vi "TCPIP RED WRITE.vi"() -> ()   [LabVIEW 2015]
uses:
  Galobal variable_TI.vi
panel:
  out "NG":bool
  out "Ok":bool
  out "loop Itration":i32
  out "Coordinate":string
  out "Data Read":string
  out "substring":string
  in  "Data Write":string
  out "data out 2":string
  out "error out 3":errorcluster
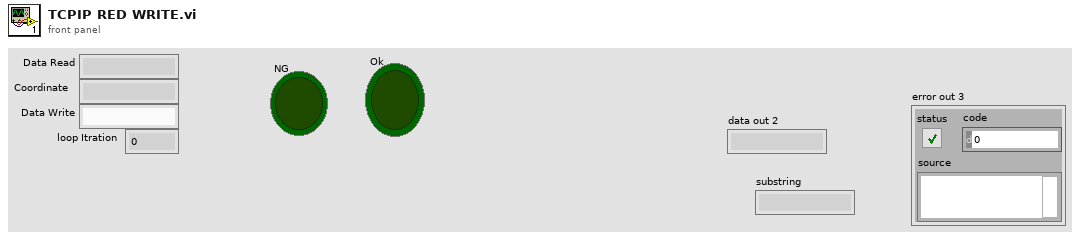
[diagram p1: front panel]
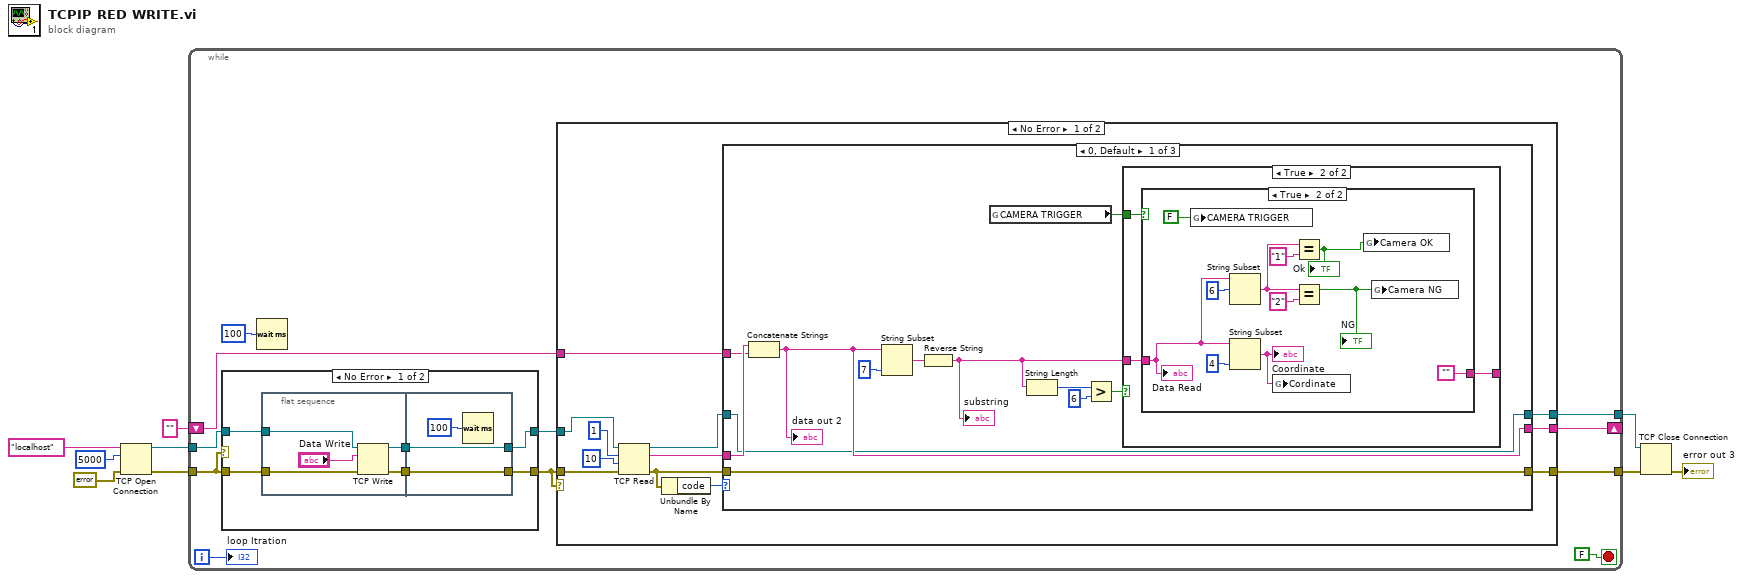
[diagram p0: block diagram]
diagram:
  n1 = TCP Open Connection(address="localhost", remote port or service name=u16 5000, error in (no error)=errorcluster {"status"=FALSE, "code"=0, "source"=""}) -> (connection ID=w3:refnum<k5>, error out=w2:errorcluster)  [unwired: 2 in]
  n2 = while {
    tunnel: [w18] -> w8
    tunnel: [w17] -> w7
    tunnel: w3 -> [w14]
    tunnel: w2 -> [w11]
    shift-right: [w15] -> _
    shift-left: "" -> [w16]
    i -> [w10]
    stop <- FALSE stop-if-true
    n3 = case shown="No Error" w11 {
      tunnel: w14 -> [w26 w36]
      tunnel: w11 -> [w25 w35]
      tunnel: [w24 w36] -> w12
      tunnel: [w23 w35] -> w13
      frame No Error {
        n4 = flat-sequence {
          tunnel: w26 -> [w31]
          tunnel: w25 -> [w30]
          tunnel: [w29] -> w22
          tunnel: [w28] -> w21
          tunnel: [w33] -> w23
          tunnel: [w34] -> w24
          tunnel: w22 -> [w34]
          tunnel: w21 -> [w33]
          frame #0 {
            n5 = TCP Write(connection ID=w31, data in="Data Write", error in (no error)=w30) -> (connection ID out=w29:refnum<k5>, error out=w28:errorcluster)  [unwired: 1 in, 1 out]
          }
          frame #1 {
            n6 = Wait (ms)(milliseconds to wait=u32 100) -> ()  [unwired: 1 out]
          }
        }
      }
      frame Error {
      }
    }
    n7 = Wait (ms)(milliseconds to wait=u32 100) -> ()  [unwired: 1 out]
    n8 = case shown="No Error" w13 {
      tunnel: [w39 w83] -> w18
      tunnel: [w37 w82] -> w17
      tunnel: w12 -> [w46 w83]
      tunnel: w13 -> [w45 w82]
      tunnel: w16 -> [w43 w81]
      tunnel: [w42 w81] -> w15
      frame No Error {
        n9 = TCP Read(connection ID=w46, bytes to read=1, error in (no error)=w45, 9:10 ("timeout ms (25000)")) -> (connection ID out=w40:refnum<k5>, data out=w44:string, error out=w38:errorcluster)  [unwired: 1 in]
        n10 = Unbundle By Name(w38) -> ("code"=w41:i32)
        n11 = case shown="0, Default" w41 {
          tunnel: w44 -> [w60 _ w79]
          tunnel: w43 -> [w59 w78 _]
          tunnel: [w58 w78 w79] -> w42
          tunnel: [w50 w77 w80] -> w39
          tunnel: w40 -> [w50 w77 w80]
          tunnel: w38 -> [w49 _ _]
          tunnel: [w49 _ _] -> w37
          frame 0, Default {
            n12 = Concatenate Strings(w60, w59) -> (w58:string)
            "data out 2" <- w58
            n13 = String Subset(string=w58, length (rest)=7 ("length (rest)")) -> (substring=w56:string)  [unwired: 1 in]
            n14 = Reverse String(1:w56) -> (0:w51:string)
            "substring" <- w51
            n15 = global read "Galobal variable_TI.vi" "CAMERA TRIGGER"() -> (w53:bool)
            n16 = String Length(string=w51) -> (length=w55:i32)
            n17 = Greater?(x=w55, y=6) -> (0:w54:bool)
            n18 = case shown="True" w54 {
              tunnel: w53 -> [_ w64]
              tunnel: w51 -> [w61 w63]
              tunnel: [w61 w62] -> _
              frame False {
              }
              frame True {
                n19 = case shown="True" w64 {
                  tunnel: w63 -> [w65 w67]
                  tunnel: [w65 ""] -> w62
                  frame False {
                  }
                  frame True {
                    n20 = global write "Galobal variable_TI.vi" "CAMERA TRIGGER"(FALSE ("CAMERA TRIGGER")) -> ()
                    n21 = String Subset(string=w67, offset (0)=6) -> (substring=w70:string)  [unwired: 1 in]
                    n22 = String Subset(string=w67, length (rest)=4 ("length (rest)")) -> (substring=w76:string)  [unwired: 1 in]
                    "Coordinate" <- w76
                    n23 = global write "Galobal variable_TI.vi" "Cordinate"(w76) -> ()
                    n24 = Equal?(x=w70, y="1") -> (x = y?=w69:bool)
                    "Ok" <- w69
                    n25 = Equal?(x=w70, y="2") -> (x = y?=w68:bool)
                    "NG" <- w68
                    n26 = global write "Galobal variable_TI.vi" "Camera OK"(w69) -> ()
                    n27 = global write "Galobal variable_TI.vi" "Camera NG"(w68) -> ()
                    "Data Read" <- w67
                  }
                }
              }
            }
          }
          frame 1 {
          }
          frame 56 {
          }
        }
      }
      frame Error {
      }
    }
    "loop Itration" <- w10
  }
  n28 = TCP Close Connection(connection ID=w8, error in (no error)=w7) -> (error out=→"error out 3":errorcluster)  [unwired: 1 in, 1 out]
